vi "Write Tempo de espera.vi"(8 "error in (no error)":errorcluster, 10 "Tempo de espera":u16, 11 "CCDCamera in":refnum<class "Simulated_CCD_Camera.lvclass">) -> (0 "error out":errorcluster, 3 "CCDCamera out":refnum<class "Simulated_CCD_Camera.lvclass">)   [LabVIEW 2018, in "Simulated_CCD_Camera.lvclass"]
uses:
  Simulated_CCD_Camera.lvclass
  Simulated_CCD_Camera.lvclass/Simulated_CCD_Camera.ctl
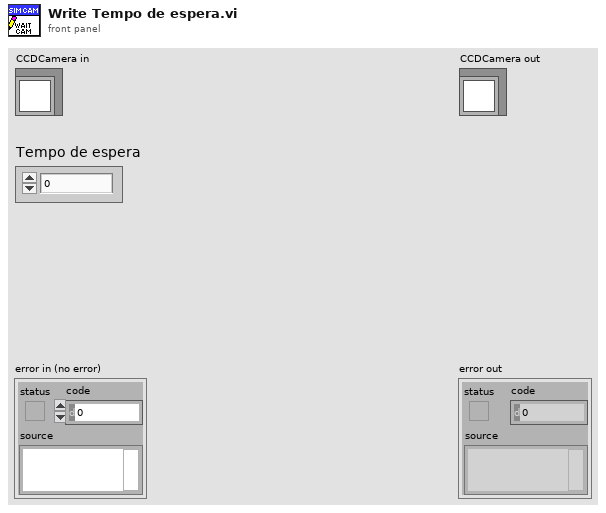
[diagram p1: front panel]
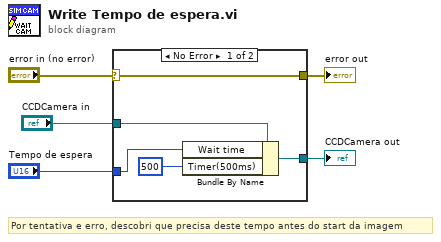
[diagram p0: block diagram]
diagram:
  # "Por tentativa e erro, descobri que precisa deste tempo antes do start da imagem"
  n1 = case shown="No Error" "error in (no error)" {
    selector: "error in (no error)" -> [w10 w11]
    tunnel: [w10 w11] -> w4
    tunnel: [w8 w12] -> w2
    tunnel: "CCDCamera in" -> [w9 w12]
    tunnel: "Tempo de espera" -> [w7 _]
    frame No Error {
      n2 = Bundle By Name(cluster=w9, "Wait time"=w7, "Timer(500ms)"=u16 500) -> (w8:refnum<class "Simulated_CCD_Camera.lvclass">)
    }
    frame Error {
    }
  }
  "error out" <- w4
  "CCDCamera out" <- w2
